vi "Periodic Tasks.vi"(8 "error in":errorcluster) -> ()   [LabVIEW 2011]
doc: "This VI runs in parallel to other tasks. It can contain as many user-defined periodic loops as you need. These can carry out PID or other sorts of timed response."
uses:
  <vilib>/Rock Robotics/WPI/Ultrasonic/WPI_UltrasonicRangeUnits.ctl
  <vilib>/Rock Robotics/SystemInterfaces/Utilities/FPGA_UtilitiesLED State.ctl
  <vilib>/Rock Robotics/SystemInterfaces/Utilities/FPGA_UtilitiesLED Source.ctl
  Robot Global Data.vi
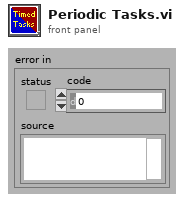
[diagram p1: front panel]
types:
  T1 = typedef "WPI_DigitalInputDevRef.ctl" = cluster{"DevStatus":errorcluster, "DIO Channel":T2, "Digital Module":T3}
  T2 = typedef "FPGA_DIOChannel.ctl" = enum8{"DIO 1", "DIO 2", "DIO 3", "DIO 4", "DIO 5", "DIO 6", "DIO 7", "DIO 8", "DIO 9", "DIO 10", "DIO 11", "DIO 12", "DIO 13", "DIO 14", "Invalid"}
  T3 = typedef "FPGA_TypedefDigitalModule.ctl" = enum16{"Digital Module 1", "Digital Module 2"}
  T4 = typedef "WPI_MotorControlDeviceRef.ctl" = cluster{"DeviceStatus":errorcluster, "Type":enum16{"PWM", "CAN"}, "PWM":cluster{"Digital Module":T3, "PWM Channel":T5, "DeadBand":T6}, "CAN":cluster{"Device Number":u8, "Control Mode":T7, "Semaphore":T8, "Max Vout":dbl}, "Invert":bool, "TransformRef":T9, "InvTransformRef":T9}
  T5 = typedef "FPGA_DIOPWMChannel.ctl" = enum8{"PWM 1", "PWM 2", "PWM 3", "PWM 4", "PWM 5", "PWM 6", "PWM 7", "PWM 8", "PWM 9", "PWM 10", "Invalid"}
  T6 = typedef "WPI_PWMDeadband.ctl" = cluster{"Name":string, "maxPositivePwm":i32, "minPositivePwm":i32, "centerPwm":i32, "maxNegativePwm":i32, "minNegativePwm":i32, "angularRange":u16}
  T7 = typedef "WPI_CANJaguar_ControlMode.ctl" = enum8{"Percent VBus", "Current", "Speed", "Position", "Voltage"}
  T8 = typedef "Semaphore RefNum" = refnum<k1>
  T9 = typedef "WPI_PWMTransform_ConPane.ctl" = refnum<vi>
  T10 = typedef "WPI_EncoderDevRef.ctl" = cluster{"DevStatus":errorcluster, "EncoderIndex":T11, "CounterIndex":T12, "DistancePerCount":dbl, "Decoding Type":T13}
  T11 = typedef "FPGA_EncoderIdx.ctl" = enum8{"Enc 0", "Enc 1", "Enc 2", "Enc 3", "Invalid"}
  T12 = typedef "FPGA_CounterCtrSystemIndex.ctl" = enum8{"Ctr 0", "Ctr 1", "Ctr 2", "Ctr 3", "Ctr 4", "Ctr 5", "Ctr 6", "Ctr 7", "Invalid"}
  T13 = typedef "WPI_EncoderType.ctl" = enum16{"1x", "2x", "4x"}
  T14 = typedef "WPI_UltrasonicDeviceRef.ctl" = cluster{"DevStatus":errorcluster, "Ping Digital Module":T3, "Echo Digital Module":T3, "Ping Channel":T2, "Echo Channel":T2, "CntIndex":T12}
  T15 = typedef "WPI_AnalogChannelDevRef.ctl" = cluster{"DevStatus":errorcluster, "Analog Module":T16, "Analog Channel":T17}
  T16 = typedef "FPGA_TypedefAnalogModule.ctl" = enum16{"Analog Module 1", "Analog Module 2"}
  T17 = typedef "FPGA_AIChannel.ctl" = enum8{"AI 1", "AI 2", "AI 3", "AI 4", "AI 5", "AI 6", "AI 7", "AI 8", "Invalid"}
  T18 = typedef "WPI_RobotDriveDevRef.ctl" = cluster{"DevStatus":errorcluster, "Motors[]":T4[], "Square Inputs":bool, "Max Output":dbl, "Isochronous":bool}
  T19 = typedef "FPGA_UtilitiesLED State.ctl" = enum16{"Off", "On", "Toggle"}
  T20 = typedef "FPGA_UtilitiesLED Source.ctl" = enum16{"User LED", "FPGA LED"}
  T21 = typedef "WPI_UltrasonicRangeUnits.ctl" = enum16{"inches", "mm"}
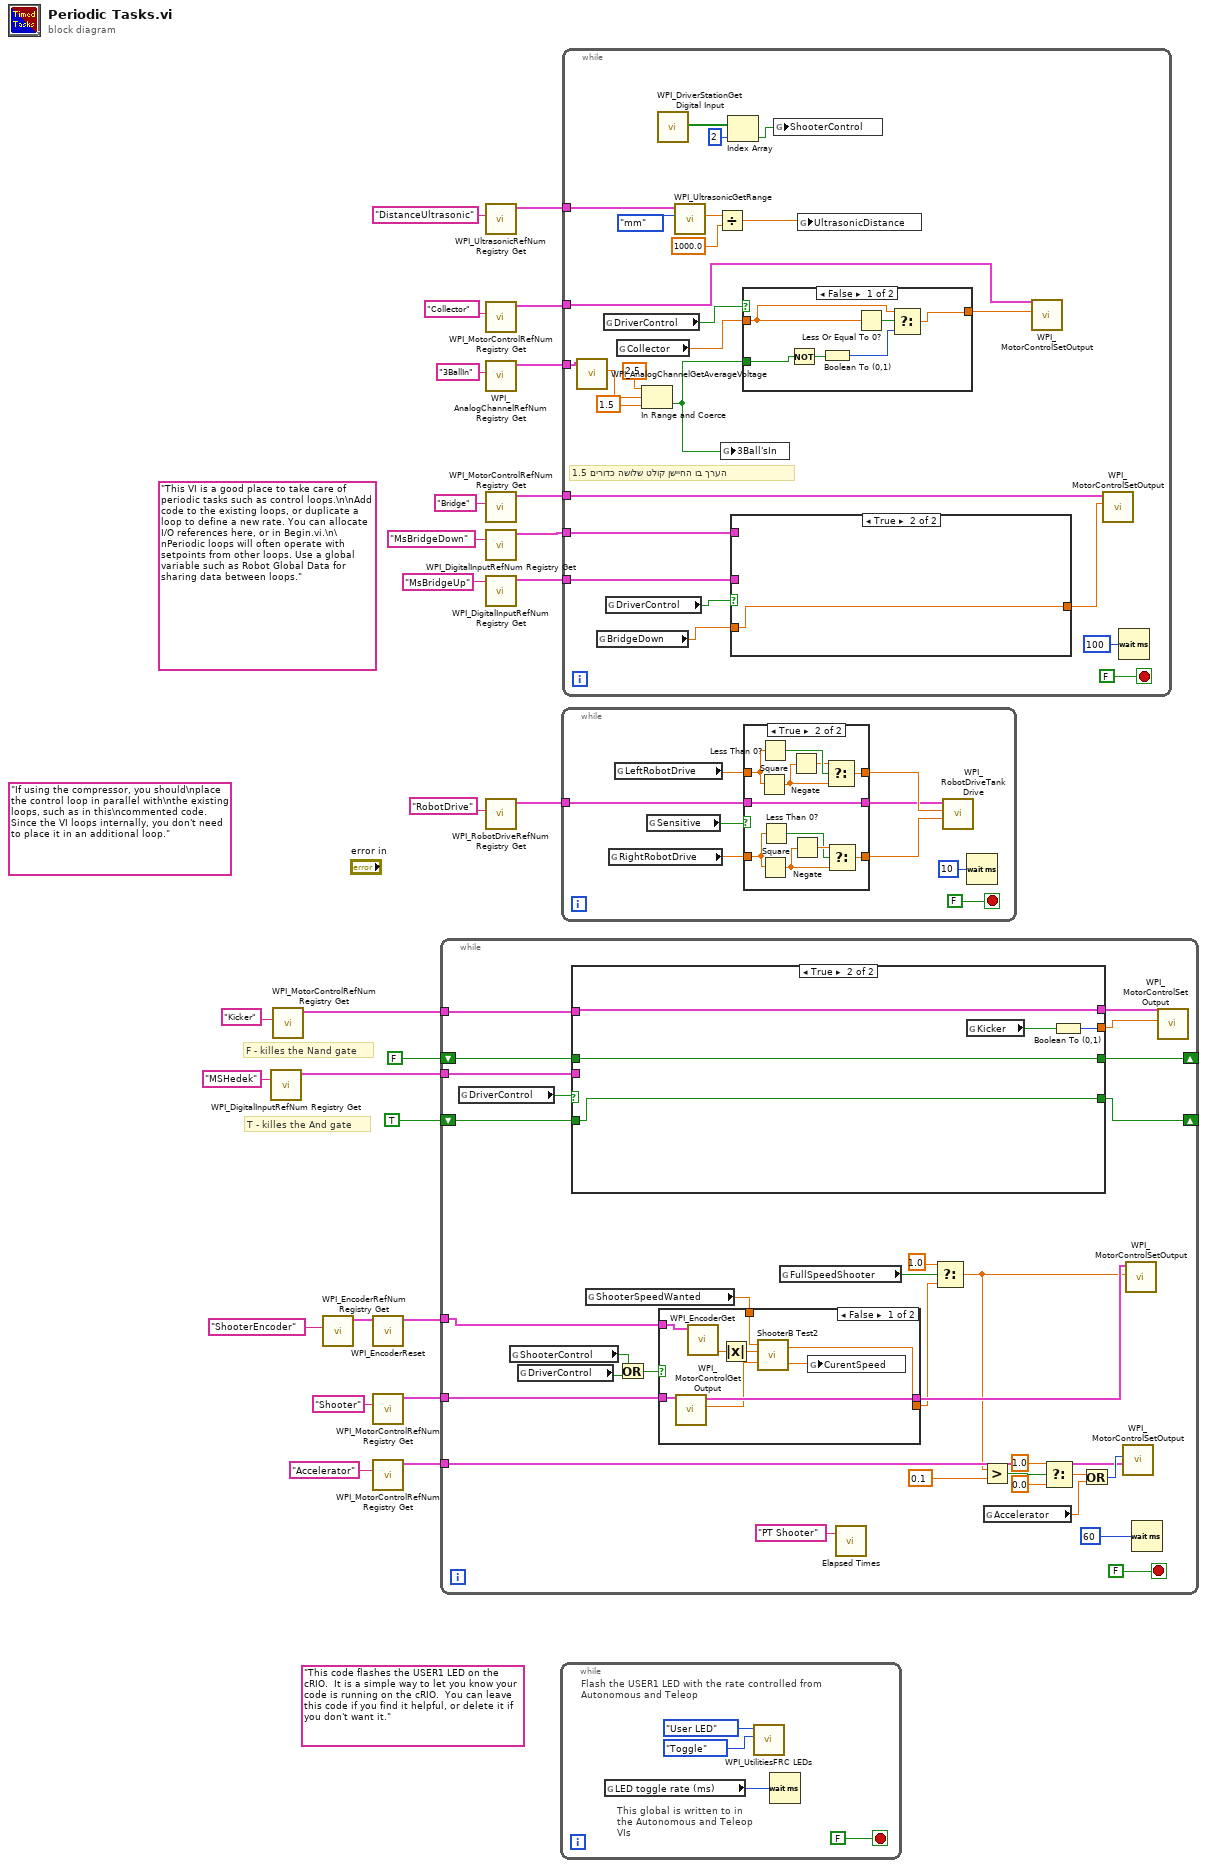
[diagram p0: block diagram]
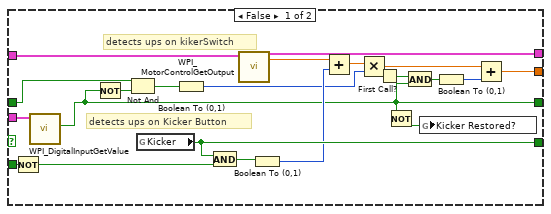
[diagram p2: hidden frame]
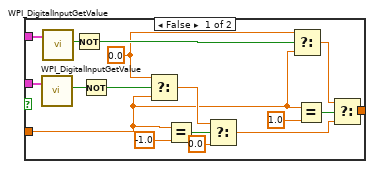
[diagram p6: hidden frame]
diagram:
  (unwired) "If using the compressor, you should\nplace the control loop in parallel with\nthe existing loops, such as in this\ncommented code. Since the VI loops internally, you don't need to place it in an additional loop."
  (unwired) "This code flashes the USER1 LED on the cRIO.  It is a simple way to let you know your code is running on the cRIO.  You can leave this code if you find it helpful, or delete it if you don't want it."
  (unwired) "This VI is a good place to take care of periodic tasks such as control loops.\n\nAdd code to the existing loops, or duplicate a loop to define a new rate. You can allocate I/O references here, or in Begin.vi.\n\nPeriodic loops will often operate with setpoints from other loops. Use a global variable such as Robot Global Data for sharing data between loops."
  # "T - killes the And gate"
  # "F - killes the Nand gate"
  n1 = call <vilib>:"WPI_DigitalInputRefNum Registry Get.vi"("refnum name"="MSHedek") -> ("DigitalInputDevRef"=w12:T1)  [unwired: 9 in, 1 out]
  n2 = call <vilib>:"WPI_MotorControlRefNum Registry Get.vi"("refnum name"="Kicker") -> ("MotorControlDevRef"=w13:T4)  [unwired: 9 in, 1 out]
  n3 = call <vilib>:"WPI_EncoderRefNum Registry Get.vi"("refnum name"="ShooterEncoder") -> ("EncoderDevRef"=w9:T10)  [unwired: 9 in, 1 out]
  n4 = call <vilib>:"WPI_EncoderReset.vi"("EncoderDevRef"=w9) -> ("EncoderDevRef"=w6:T10)  [unwired: 9 in, 1 out]
  n5 = call <vilib>:"WPI_MotorControlRefNum Registry Get.vi"("refnum name"="Shooter") -> ("MotorControlDevRef"=w5:T4)  [unwired: 9 in, 1 out]
  n6 = call <vilib>:"WPI_MotorControlRefNum Registry Get.vi"("refnum name"="Accelerator") -> ("MotorControlDevRef"=w1:T4)  [unwired: 9 in, 1 out]
  n7 = while {
    tunnel: w13 -> [w48]
    tunnel: w12 -> [w47]
    shift-right: [w38] -> _
    shift-left: FALSE ("Value") -> [w56]
    shift-right: [w54] -> _
    shift-left: TRUE ("Kicker") -> [w37]
    tunnel: w6 -> [w52]
    tunnel: w5 -> [w51]
    tunnel: w1 -> [w39]
    stop <- FALSE stop-if-true
    n8 = global read "Robot Global Data.vi" "DriverControl"() -> (w36:bool)
    n9 = global read "Robot Global Data.vi" "ShooterControl"() -> (w30:bool)
    n10 = global read "Robot Global Data.vi" "DriverControl"() -> (w29:bool)
    n11 = case shown="True" w36 {
      tunnel: w56 -> [w79 w81]
      tunnel: [w77 w83] -> w55
      tunnel: [w75 w80] -> w54
      tunnel: w37 -> [w74 w80]
      tunnel: [w70 w84] -> w53
      tunnel: w48 -> [w64 w83]
      tunnel: w47 -> [w61 _]
      tunnel: [w60 w81] -> w38
      frame False {
        # "detects ups on Kicker Button"
        # "detects ups on kikerSwitch"
        n12 = Not(x=w74) -> (.not. x?=w73:bool)
        n13 = call <vilib>:"WPI_DigitalInputGetValue.vi"("DigitalInputDevRef"=w61) -> ("Value"=w60:bool)  [unwired: 8 in, 2 out]
        n14 = Not(x=w60) -> (.not. x?=w78:bool)
        n15 = Not And(1:w78, 2:w79) -> (0:w76:bool)
        n16 = global read "Robot Global Data.vi" "Kicker"() -> (w75:bool)
        n17 = Boolean To (0,1)(Boolean=w76) -> (0, 1=w65:i16)
        n18 = And(x=w75, y=w73) -> (x .and. y?=w72:bool)
        n19 = call <vilib>:"WPI_MotorControlGetOutput.vi"("MotorControlDevRef"=w64) -> ("Output"=w62:dbl, "MotorControlDevRef"=w77:T4)  [unwired: 8 in, 1 out]
        n20 = Boolean To (0,1)(Boolean=w72) -> (0, 1=w67:i16)
        n21 = Add(x=w62, y=w67) -> (x+y=w66:dbl)
        n22 = Multiply(x=w66, y=w65) -> (x*y=w63:dbl)
        n23 = First Call?() -> (First Call?: T/F=w71:bool)
        n24 = Not(x=w60) -> (.not. x?=w59:bool)
        n25 = And(x=w71, y=w60) -> (x .and. y?=w69:bool)
        n26 = global write "Robot Global Data.vi" "Kicker Restored?"(w59) -> ()
        n27 = Boolean To (0,1)(Boolean=w69) -> (0, 1=w68:i16)
        n28 = Add(x=w63, y=w68) -> (x+y=w70:dbl)
      }
      frame True {
        n29 = global read "Robot Global Data.vi" "Kicker"() -> (w82:bool)
        n30 = Boolean To (0,1)(Boolean=w82) -> (0, 1=w84:i16)
      }
    }
    n31 = global read "Robot Global Data.vi" "ShooterSpeedWanted"() -> (w50:dbl)
    n32 = Or(x=w30, y=w29) -> (x .or. y?=w28:bool)
    n33 = case shown="False" w28 {
      tunnel: w52 -> [w93 _]
      tunnel: w51 -> [w92 w94]
      tunnel: w50 -> [w90 w95]
      tunnel: [w91 w94] -> w49
      tunnel: [w89 w95] -> w33
      frame False {
        n34 = call <vilib>:"WPI_MotorControlGetOutput.vi"("MotorControlDevRef"=w92) -> ("Output"=w86:dbl, "MotorControlDevRef"=w91:T4)  [unwired: 8 in, 1 out]
        n35 = call <vilib>:"WPI_EncoderGet.vi"("EncoderDevRef"=w93) -> ("Rate"=w88:dbl)  [unwired: 5 in, 5 out]
        n36 = Absolute Value(x=w88) -> (abs(x)=w87:dbl)
        n37 = call "ShooterB Test2.vi"("GetMotorOut"=w86, "Encoder"=w87, "Shooter"=w90) -> ("CurrentSpeed"=w85:dbl, "ToMotor"=w89:dbl)
        n38 = global write "Robot Global Data.vi" "CurentSpeed"(w85) -> ()
      }
      frame True {
      }
    }
    n39 = global read "Robot Global Data.vi" "FullSpeedShooter"() -> (w35:bool)
    n40 = call "Elapsed Times.vi"("Call Name"="PT Shooter") -> ()  [unwired: 2 in, 1 out]
    n41 = Select(t=1.0, s=w35, f=w33) -> (s? t:f=w32:dbl)
    n42 = Greater?(x=w32, y=0.1 ("x")) -> (0:w45:bool)
    n43 = global read "Robot Global Data.vi" "Accelerator"() -> (w42:dbl)
    n44 = Select(t=1.0, s=w45, f=0.0) -> (s? t:f=w41:dbl)
    n45 = Or(x=w41, y=w42) -> (x .or. y?=w40:i32)
    n46 = call <vilib>:"WPI_MotorControlSetOutput.vi"("Output"=w40, "MotorControlDevRef"=w39) -> ()  [unwired: 8 in, 2 out]
    n47 = call <vilib>:"WPI_MotorControlSetOutput.vi"("Output"=w32, "MotorControlDevRef"=w49) -> ()  [unwired: 8 in, 2 out]
    n48 = Wait (ms)(milliseconds to wait=u32 60) -> ()  [unwired: 1 out]
    n49 = call <vilib>:"WPI_MotorControlSetOutput.vi"("Output"=w53, "MotorControlDevRef"=w55) -> ()  [unwired: 8 in, 2 out]
  }
  n50 = call <vilib>:"WPI_UltrasonicRefNum Registry Get.vi"("refnum name"="DistanceUltrasonic") -> ("UltrasonicDevRef"=w3:T14)  [unwired: 9 in, 1 out]
  n51 = call <vilib>:"WPI_MotorControlRefNum Registry Get.vi"("refnum name"="Collector") -> ("MotorControlDevRef"=w19:T4)  [unwired: 9 in, 1 out]
  n52 = call <vilib>:"WPI_AnalogChannelRefNum Registry Get.vi"("refnum name"="3BallIn") -> ("AIDeviceRef"=w18:T15)  [unwired: 9 in, 1 out]
  n53 = call <vilib>:"WPI_MotorControlRefNum Registry Get.vi"("refnum name"="Bridge") -> ("MotorControlDevRef"=w24:T4)  [unwired: 9 in, 1 out]
  n54 = call <vilib>:"WPI_DigitalInputRefNum Registry Get.vi"("refnum name"="MsBridgeDown") -> ("DigitalInputDevRef"=w23:T1)  [unwired: 9 in, 1 out]
  n55 = call <vilib>:"WPI_DigitalInputRefNum Registry Get.vi"("refnum name"="MsBridgeUp") -> ("DigitalInputDevRef"=w22:T1)  [unwired: 9 in, 1 out]
  n56 = call <vilib>:"WPI_RobotDriveRefNum Registry Get.vi"("refnum name"="RobotDrive") -> ("RobotDriveDevRef"=w16:T18)  [unwired: 9 in, 1 out]
  n57 = while {
    stop <- FALSE stop-if-true
    # "This global is written to in the Autonomous and Teleop VIs"
    # "Flash the USER1 LED with the rate controlled from Autonomous and Teleop"
    n58 = global read "Robot Global Data.vi" "LED toggle rate (ms)"() -> (w96:u32)
    n59 = call <vilib>:"WPI_UtilitiesFRC LEDs.vi"("State"=FPGA_UtilitiesLED_State."Toggle", "LED Type"=FPGA_UtilitiesLED_Source."User LED") -> ()  [unwired: 1 in, 9 out]
    n60 = Wait (ms)(milliseconds to wait=w96) -> ()  [unwired: 1 out]
  }
  n61 = while {
    tunnel: w16 -> [w100]
    stop <- FALSE stop-if-true
    n62 = global read "Robot Global Data.vi" "RightRobotDrive"() -> (w106:dbl)
    n63 = global read "Robot Global Data.vi" "LeftRobotDrive"() -> (w105:dbl)
    n64 = global read "Robot Global Data.vi" "Sensitive"() -> (w104:bool)
    n65 = case shown="True" w104 {
      tunnel: w106 -> [w110 w121]
      tunnel: w105 -> [w111 w117]
      tunnel: [w111 w115] -> w103
      tunnel: [w110 w114] -> w102
      tunnel: [w109 w113] -> w101
      tunnel: w100 -> [w109 w113]
      frame False {
      }
      frame True {
        n66 = Square(x=w117) -> (x^2=w116:dbl)
        n67 = Less Than 0?(x=w117) -> (x < 0?=w122:bool)
        n68 = Square(x=w121) -> (x^2=w120:dbl)
        n69 = Less Than 0?(x=w121) -> (x < 0?=w112:bool)
        n70 = Negate(x=w116) -> (-x=w118:dbl)
        n71 = Negate(x=w120) -> (-x=w119:dbl)
        n72 = Select(t=w118, s=w122, f=w116) -> (s? t:f=w115:dbl)
        n73 = Select(t=w119, s=w112, f=w120) -> (s? t:f=w114:dbl)
      }
    }
    n74 = call <vilib>:"WPI_RobotDriveTankDrive.vi"("Right axis value"=w102, "Left axis value"=w103, "RobotDriveDevRef"=w101) -> ()  [unwired: 7 in, 2 out]
    n75 = Wait (ms)(milliseconds to wait=u32 10) -> ()  [unwired: 1 out]
  }
  n76 = while {
    tunnel: w24 -> [w145]
    tunnel: w23 -> [w144]
    tunnel: w22 -> [w143]
    tunnel: w19 -> [w141]
    tunnel: w18 -> [w142]
    tunnel: w3 -> [w136]
    stop <- FALSE stop-if-true
    # "1.5 הערך בו החיישן קולט שלושה כדורים"
    n77 = call <vilib>:"WPI_AnalogChannelGetAverageVoltage.vi"("AIDeviceRef"=w142) -> ("Voltage"=w129:dbl)  [unwired: 8 in, 2 out]
    n78 = global read "Robot Global Data.vi" "BridgeDown"() -> (w133:dbl)
    n79 = global read "Robot Global Data.vi" "DriverControl"() -> (w131:bool)
    n80 = global read "Robot Global Data.vi" "DriverControl"() -> (w134:bool)
    n81 = global read "Robot Global Data.vi" "Collector"() -> (w132:dbl)
    n82 = In Range and Coerce(upper limit=2.5 ("y"), x=w129, lower limit=1.5 ("y")) -> (In Range?=w126:bool)  [unwired: 1 out]
    n83 = call <vilib>:"WPI_DriverStationGet Digital Input.vi"() -> ("Driver Station Digital Input (1-8)"=w125:bool[])  [unwired: 11 in]
    n84 = call <vilib>:"WPI_UltrasonicGetRange.vi"("Range Units"=WPI_UltrasonicRangeUnits."mm", "UltrasonicDevRef"=w136) -> ("Distance"=w138:dbl)  [unwired: 7 in, 2 out]
    n85 = Divide(x=w138, y=1000.0) -> (x/y=w137:dbl)
    n86 = global write "Robot Global Data.vi" "3Ball'sIn"(w126) -> ()
    n87 = Index Array(array=w125, index=2) -> (element=w123:bool)
    n88 = case shown="True" w134 {
      tunnel: w144 -> [w167 _]
      tunnel: w143 -> [w166 _]
      tunnel: [w157 w172] -> w135
      tunnel: w133 -> [w155 w172]
      frame False {
        w165 = 0.0 ("t")
        n89 = call <vilib>:"WPI_DigitalInputGetValue.vi"("DigitalInputDevRef"=w166) -> ("Value"=w171:bool)  [unwired: 8 in, 2 out]
        n90 = call <vilib>:"WPI_DigitalInputGetValue.vi"("DigitalInputDevRef"=w167) -> ("Value"=w170:bool)  [unwired: 8 in, 2 out]
        n91 = Not(x=w170) -> (.not. x?=w169:bool)
        n92 = Not(x=w171) -> (.not. x?=w168:bool)
        n93 = Select(t=w165, s=w168, f=w155) -> (s? t:f=w159:dbl)
        n94 = Equal?(x=w155, y=-1.0) -> (x = y?=w160:bool)
        n95 = Select(t=w159, s=w160, f=0.0) -> (s? t:f=w158:dbl)
        n96 = Select(t=w165, s=w169, f=w155) -> (s? t:f=w162:dbl)
        n97 = Equal?(x=w155, y=1.0) -> (x = y?=w163:bool)
        n98 = Select(t=w162, s=w163, f=w158) -> (s? t:f=w157:dbl)
      }
      frame True {
      }
    }
    n99 = case shown="False" w131 {
      tunnel: w132 -> [w152 w154]
      tunnel: [w151 w154] -> w130
      tunnel: w126 -> [w148 _]
      frame False {
        n100 = Not(x=w148) -> (.not. x?=w150:bool)
        n101 = Boolean To (0,1)(Boolean=w150) -> (0, 1=w149:i16)
        n102 = Less Or Equal To 0?(x=w152) -> (x <= 0?=w153:bool)
        n103 = Select(t=w152, s=w153, f=w149) -> (s? t:f=w151:dbl)
      }
      frame True {
      }
    }
    n104 = global write "Robot Global Data.vi" "ShooterControl"(w123) -> ()
    n105 = global write "Robot Global Data.vi" "UltrasonicDistance"(w137) -> ()
    n106 = call <vilib>:"WPI_MotorControlSetOutput.vi"("Output"=w130, "MotorControlDevRef"=w141) -> ()  [unwired: 8 in, 2 out]
    n107 = call <vilib>:"WPI_MotorControlSetOutput.vi"("Output"=w135, "MotorControlDevRef"=w145) -> ()  [unwired: 8 in, 2 out]
    n108 = Wait (ms)(milliseconds to wait=u32 100) -> ()  [unwired: 1 out]
  }
